vi "Ximea Camera Messenger.vi"(0 "Notifier Name":string, 2 "Ximea Actions":T5=enum."Error Check", 5 "Ximea  Parameter":T2, 7 "ROI Setup":T1, 9 "# of Frames":u32, 11 "File Save Path":path) -> (4 "Notifier Name (Dup)":string, 6 "Running?":bool, 8 "Ximea Parameter Out":T2, 10 "Ximea ROI Out":T1, 15 "Image Ref":T4)   [LabVIEW 2021]
uses:
  Ximea Controls/Ximea Actions.ctl
  Ximea Controls/Ximea Parameters.ctl
  Ximea Controls/Ximea Parameter List.ctl
  Ximea Controls/Ximea ROI.ctl
  <vilib>/vision/Image Controls.llb/IMAQ Image.ctl
  Ximea Controls/Ximea Notifier Element.ctl
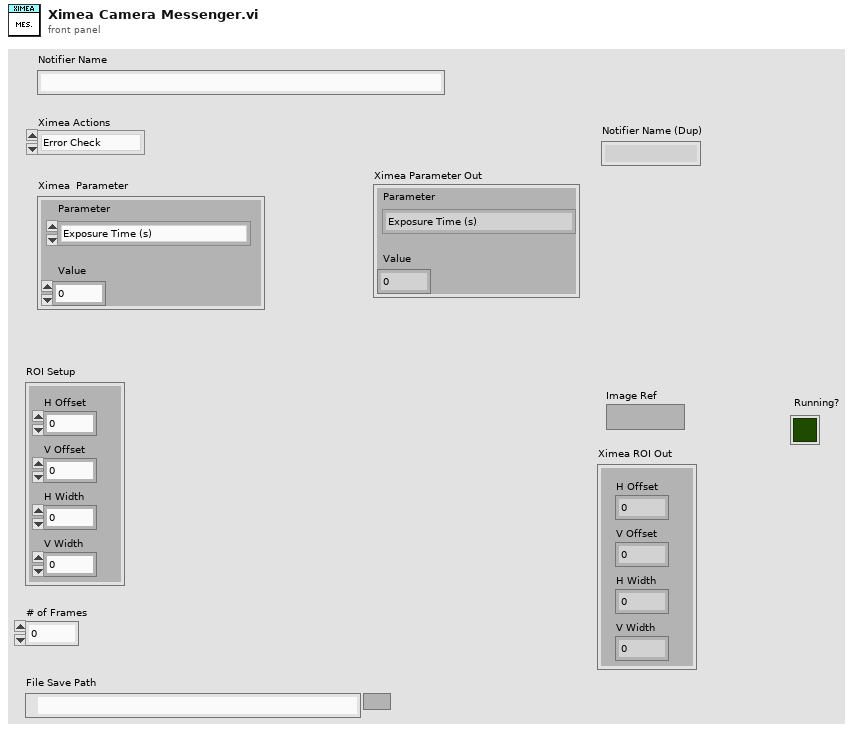
[diagram p1: front panel]
types:
  T1 = typedef "Ximea ROI.ctl" = cluster{"H Offset":i32, "V Offset":i32, "H Width":i32, "V Width":i32}
  T2 = typedef "Ximea Parameters.ctl" = cluster{"Parameter":T3, "Value":sgl}
  T3 = typedef "Ximea Parameter List.ctl" = enum16{"Exposure Time (s)", "Gain"}
  T4 = typedef "IMAQ Image.ctl" = refnum<image>
  T5 = typedef "Ximea Actions.ctl" = enum16{"Idle", "Error Check", "Preview", "Record", "Soft Trigger", "Abort", "Record Settings", "Set Parameter", "Get Parameter", "Set ROI", "Get ROI", "Status", "Quit"}
  T6 = typedef "Ximea Notifier Element.ctl" = cluster{"Ximea Actions":T5, "Received?":bool, "Ximea Parameter":T2, "Ximea ROI":T1, "Running?":bool, "File Path":path, "# of frames":u32, "Image Ref":T4, "Error":errorcluster, "Trigger?":bool, "ROI Increment":i32}
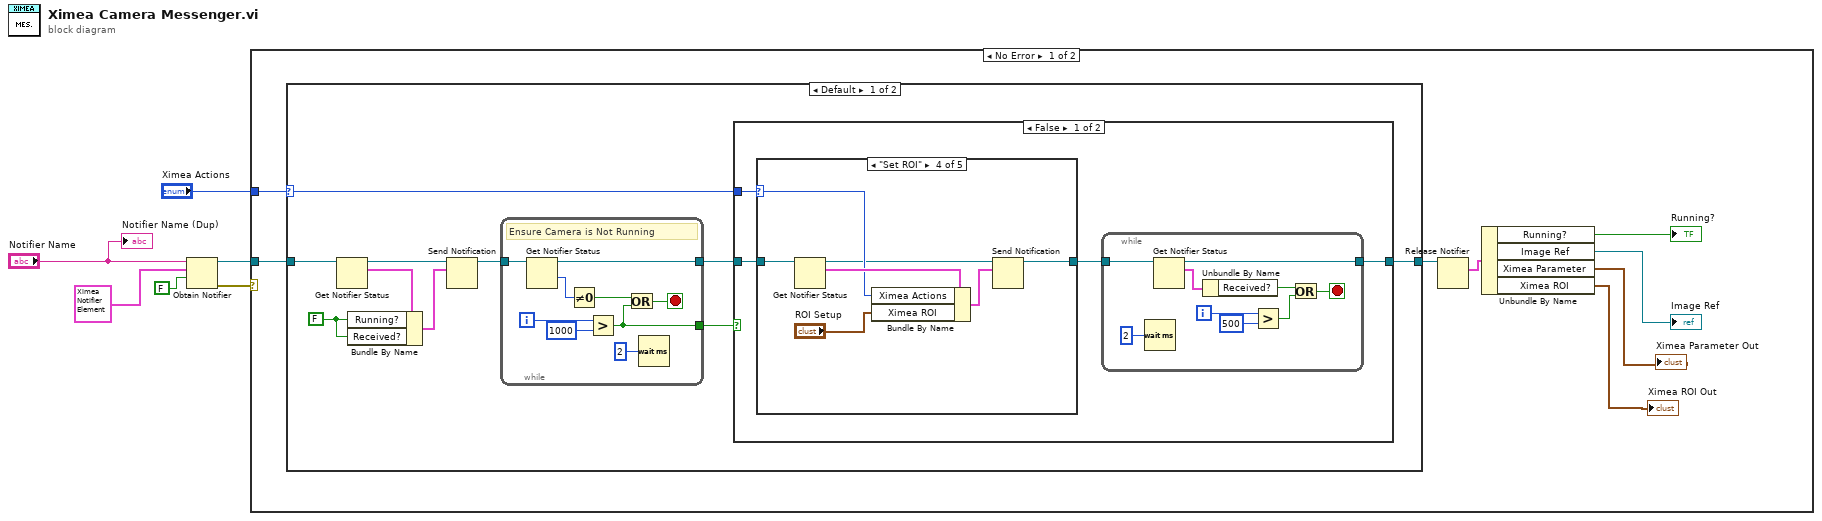
[diagram p0: block diagram]
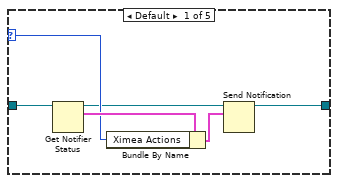
[diagram p2: hidden frame]
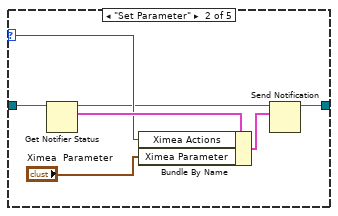
[diagram p3: hidden frame]
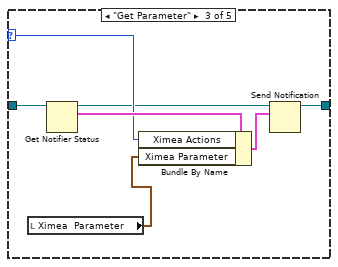
[diagram p4: hidden frame]
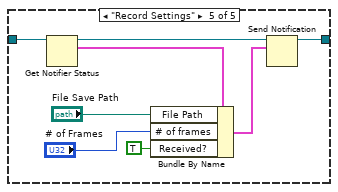
[diagram p5: hidden frame]
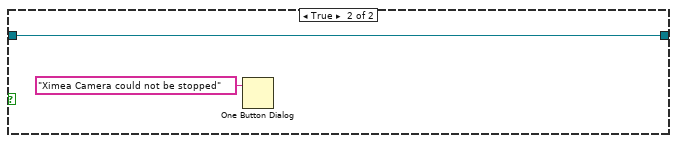
[diagram p6: hidden frame]
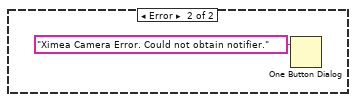
[diagram p8: hidden frame]
diagram:
  n1 = Obtain Notifier(name (unnamed)="Notifier Name", notification data type=T6 {"Ximea Actions"=enum."Quit", "Received?"=TRUE, "Ximea Parameter"={"Parameter"=enum."Exposure Time (s)", "Value"=0.0}, "Ximea ROI"={"H Offset"=0, "V Offset"=0, "H Width"=0, "V Width"=0}, "Running?"=FALSE, "File Path"=path "", "# of frames"=0, "Image Ref"=refnum, "Error"={"status"=FALSE, "code"=0, "source"=""}, "Trigger?"=FALSE, "ROI Increment"=0} ("Ximea Camera Cluster"), create if not found? (T)=FALSE) -> (notifier out=w3:refnum<notifier>, error out=w4:errorcluster)  [unwired: 1 in, 1 out]
  n2 = case shown="No Error" w4 {
    tunnel: w3 -> [w14 _]
    tunnel: "Ximea Actions" -> [w13 _]
    frame No Error {
      n3 = case shown="Default" w13 {
        selector: w13 -> [w20 _]
        tunnel: w14 -> [w24 w84]
        tunnel: [w19 w84] -> w9
        frame Default {
          w15 = FALSE ("Running?")
          n4 = Get Notifier Status(notifier=w24) -> (notifier out=w18:refnum<notifier>, current notification=w17:T6)  [unwired: 1 in, 3 out]
          n5 = Bundle By Name(cluster=w17, "Running?"=w15, "Received?"=w15) -> (w16:T6)
          n6 = Send Notification(notification=w16, notifier=w18) -> (notifier out=w23:refnum<notifier>)  [unwired: 1 in, 1 out]
          n7 = while {
            tunnel: w23 -> [w83]
            tunnel: [w82] -> w21
            tunnel: [w77] -> w22
            i -> [w79]
            stop <- w81 stop-if-true
            # "Ensure Camera is Not Running"
            n8 = Get Notifier Status(notifier=w83) -> (notifier out=w82:refnum<notifier>, # waiting=w76:i32)  [unwired: 1 in, 3 out]
            n9 = Not Equal To 0?(x=w76) -> (x != 0?=w75:bool)
            n10 = Greater?(x=w79, y=1000) -> (0:w77:bool)
            n11 = Or(x=w75, y=w77) -> (x .or. y?=w81:bool)
            n12 = Wait (ms)(milliseconds to wait=u32 2) -> ()  [unwired: 1 out]
          }
          n13 = case shown="False" w22 {
            tunnel: w21 -> [w26 w73]
            tunnel: w20 -> [w28 _]
            tunnel: [w25 w73] -> w19
            frame False {
              n14 = case shown="\"Set ROI\"" w28 {
                selector: w28 -> [w41 w48 w55 w62 _]
                tunnel: w26 -> [w43 w50 w57 w64 w72]
                tunnel: [w38 w45 w52 w59 w68] -> w27
                frame Default {
                  n15 = Get Notifier Status(notifier=w43) -> (notifier out=w40:refnum<notifier>, current notification=w42:T6)  [unwired: 1 in, 3 out]
                  n16 = Bundle By Name(cluster=w42, "Ximea Actions"=w41) -> (w39:T6)
                  n17 = Send Notification(notification=w39, notifier=w40) -> (notifier out=w38:refnum<notifier>)  [unwired: 1 in, 1 out]
                }
                frame "Set Parameter" {
                  n18 = Get Notifier Status(notifier=w50) -> (notifier out=w47:refnum<notifier>, current notification=w49:T6)  [unwired: 1 in, 3 out]
                  n19 = Bundle By Name(cluster=w49, "Ximea Actions"=w48, "Ximea Parameter"="Ximea  Parameter") -> (w46:T6)
                  n20 = Send Notification(notification=w46, notifier=w47) -> (notifier out=w45:refnum<notifier>)  [unwired: 1 in, 1 out]
                }
                frame "Get Parameter" {
                  n21 = local read "Ximea  Parameter"() -> (w51:T2)
                  n22 = Get Notifier Status(notifier=w57) -> (notifier out=w54:refnum<notifier>, current notification=w56:T6)  [unwired: 1 in, 3 out]
                  n23 = Bundle By Name(cluster=w56, "Ximea Actions"=w55, "Ximea Parameter"=w51) -> (w53:T6)
                  n24 = Send Notification(notification=w53, notifier=w54) -> (notifier out=w52:refnum<notifier>)  [unwired: 1 in, 1 out]
                }
                frame "Set ROI" {
                  n25 = Get Notifier Status(notifier=w64) -> (notifier out=w61:refnum<notifier>, current notification=w63:T6)  [unwired: 1 in, 3 out]
                  n26 = Bundle By Name(cluster=w63, "Ximea Actions"=w62, "Ximea ROI"="ROI Setup") -> (w60:T6)
                  n27 = Send Notification(notification=w60, notifier=w61) -> (notifier out=w59:refnum<notifier>)  [unwired: 1 in, 1 out]
                }
                frame "Record Settings" {
                  n28 = Get Notifier Status(notifier=w72) -> (notifier out=w70:refnum<notifier>, current notification=w71:T6)  [unwired: 1 in, 3 out]
                  n29 = Bundle By Name(cluster=w71, "File Path"="File Save Path", "# of frames"="# of Frames", "Received?"=TRUE) -> (w69:T6)
                  n30 = Send Notification(notification=w69, notifier=w70) -> (notifier out=w68:refnum<notifier>)  [unwired: 1 in, 1 out]
                }
              }
              n31 = while {
                tunnel: w27 -> [w37]
                tunnel: [w29] -> w25
                i -> [w34]
                stop <- w30 stop-if-true
                n32 = Wait (ms)(milliseconds to wait=u32 2) -> ()  [unwired: 1 out]
                n33 = Get Notifier Status(notifier=w37) -> (notifier out=w29:refnum<notifier>, current notification=w36:T6)  [unwired: 1 in, 3 out]
                n34 = Unbundle By Name(w36) -> ("Received?"=w35:bool)
                n35 = Greater?(x=w34, y=500) -> (0:w32:bool)
                n36 = Or(x=w35, y=w32) -> (x .or. y?=w30:bool)
              }
            }
            frame True {
              n37 = One Button Dialog(message="Ximea Camera could not be stopped") -> ()  [unwired: 1 in, 1 out]
            }
          }
        }
        frame "Status" {
        }
      }
      n38 = Release Notifier(notifier=w9) -> (last notification=w8:T6)  [unwired: 2 in, 2 out]
      n39 = Unbundle By Name(w8) -> ("Running?"=→"Running?":bool, "Image Ref"=→"Image Ref":T4, "Ximea Parameter"=→"Ximea Parameter Out":T2, "Ximea ROI"=→"Ximea ROI Out":T1)
    }
    frame Error {
      n40 = One Button Dialog(message="Ximea Camera Error. Could not obtain notifier.") -> ()  [unwired: 1 in, 1 out]
    }
  }
  "Notifier Name (Dup)" <- "Notifier Name"
